vi "Add Slave Histogram Entry.vi"(8 "error in (no error)":errorcluster, 10 "Event":T1, 11 "Controller in":refnum<class "Controller.lvclass">) -> (0 "error out":errorcluster, 3 "Controller out":refnum<class "Controller.lvclass">)   [LabVIEW 2019, in "Controller.lvlib" / "Controller.lvclass"]
uses:
  Controller.lvclass
  <vilib>/Utility/miscctls.llb/LVMapReplaceAction.ctl
  Sensors/Detector/Event.ctl
  Sensors/Detector/Muon Detector.lvclass
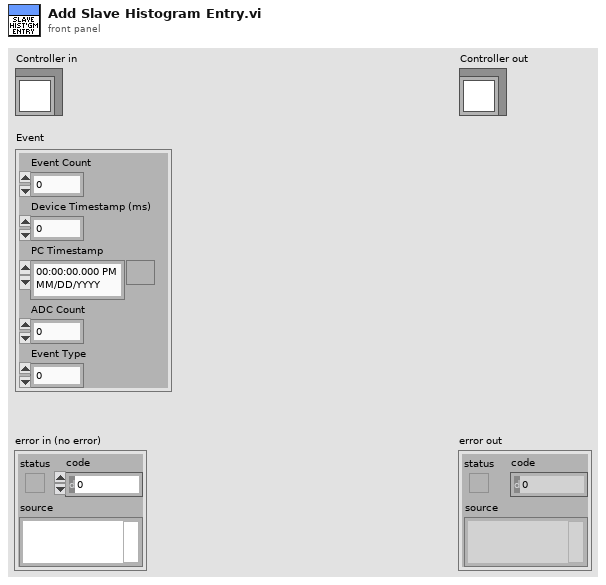
[diagram p1: front panel]
types:
  T1 = typedef "Muon Detector.lvclass/Event.ctl" = cluster{"Event Count":i32, "Device Timestamp (ms)":i32, "PC Timestamp":timestamp, "ADC Count":i32, "Event Type":u8}
  T2 = typedef "LVMapReplaceAction.ctl" = enum32{"Modify Entry only if found", "Add or Modify Entry", "Delete Entry"}
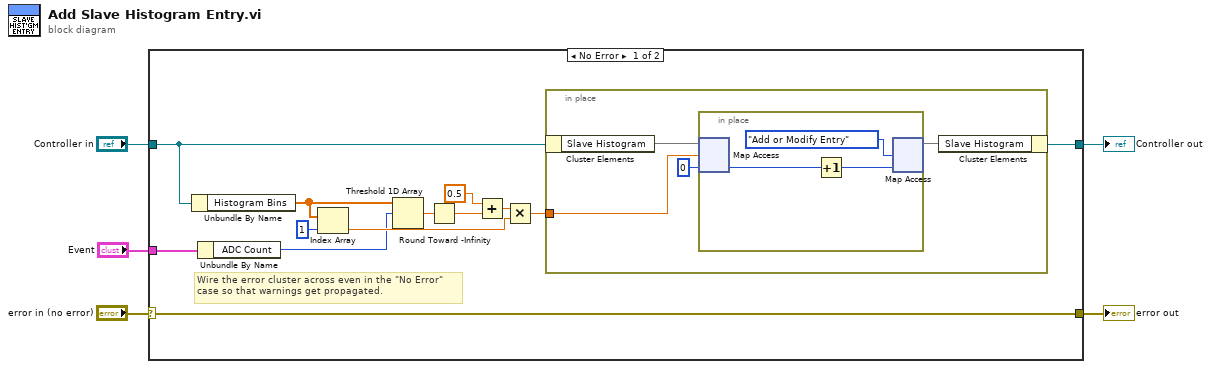
[diagram p0: block diagram]
diagram:
  n1 = case shown="No Error" "error in (no error)" {
    selector: "error in (no error)" -> [w18 w27]
    tunnel: [w18 w27] -> w4
    tunnel: [w7 w26] -> w2
    tunnel: "Controller in" -> [w6 w26]
    tunnel: "Event" -> [w10 _]
    frame No Error {
      # "Wire the error cluster across even in the \"No Error\"\ncase so that warnings get propagated."
      n2 = Unbundle By Name(w6) -> ("Histogram Bins"=w17:dbl[])
      n3 = Unbundle By Name(w10) -> ("ADC Count"=w9:i32)
      n4 = Index Array(array=w17, index=1) -> (element=w16:dbl)
      n5 = Threshold 1D Array(2:w9, 3:w17) -> (0:w15:dbl)  [unwired: 1 in]
      n6 = Round Toward -Infinity(1:w15) -> (0:w14:dbl)
      n7 = Add(x=0.5, y=w14) -> (x+y=w13:dbl)
      n8 = Multiply(x=w13, y=w16) -> (x*y=w8:dbl)
      n9 = in-place {
        in-place-border: w8 -> [w19]
        n10 = in-place-cluster #1(w6) -> ("Slave Histogram"=w22:map{dbl, i32})
        n11 = in-place {
          n12 = in-place-map #2(w22, w19, 0) -> (w24:i32)  [unwired: 1 out]
          n13 = Increment(x=w24) -> (x+1=w23:i32)
          n14 = in-place-map #2(w23, LVMapReplaceAction."Add or Modify Entry" ("action")) -> (w21:map{dbl, i32})  [unwired: 2 out]
        }
        n15 = in-place-cluster #1("Slave Histogram"=w21) -> (w7:refnum<class "Controller.lvclass">)
      }
    }
    frame Error {
    }
  }
  "error out" <- w4
  "Controller out" <- w2
